vi "takeOrder.vi"(8 "error in (no error)":errorcluster, 10 "Order.lvclass":refnum<class "Order.lvclass">, 11 "Broker in":refnum<class "Broker.lvclass">) -> (0 "error out":errorcluster, 3 "Broker out":refnum<class "Broker.lvclass">)   [LabVIEW 2016, in "Broker.lvclass"]
uses:
  Broker.lvclass
  Order Class/Order.lvclass
  Broker.lvclass/Broker.ctl
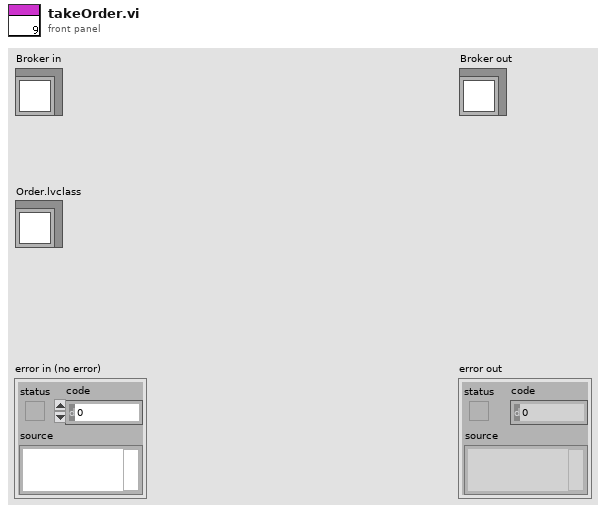
[diagram p1: front panel]
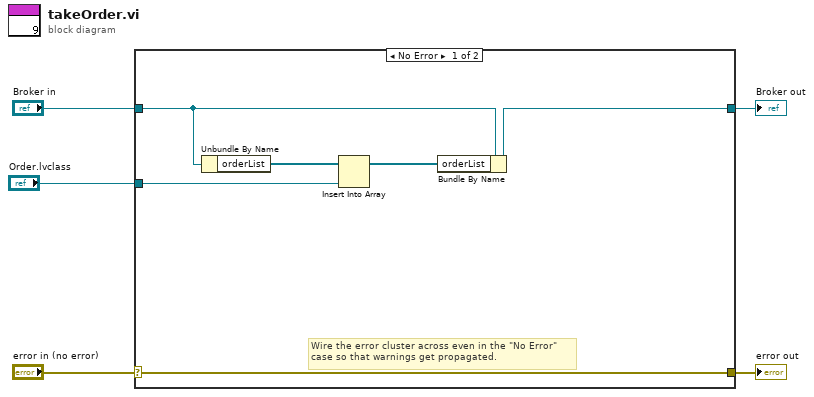
[diagram p0: block diagram]
diagram:
  n1 = case shown="No Error" "error in (no error)" {
    selector: "error in (no error)" -> [w11 w13]
    tunnel: [w11 w13] -> w4
    tunnel: [w9 w12] -> w2
    tunnel: "Broker in" -> [w10 w12]
    tunnel: "Order.lvclass" -> [w6 _]
    frame No Error {
      # "Wire the error cluster across even in the \"No Error\"\ncase so that warnings get propagated."
      n2 = Unbundle By Name(w10) -> ("orderList"=w8:refnum<class "Order.lvclass">[])
      n3 = Insert Into Array(array=w8, new element=w6) -> (w7:refnum<class "Order.lvclass">[])  [unwired: 1 in]
      n4 = Bundle By Name(cluster=w10, "orderList"=w7) -> (w9:refnum<class "Broker.lvclass">)
    }
    frame Error {
    }
  }
  "error out" <- w4
  "Broker out" <- w2
